vi "Read Teller.vi"(11 "Start Msg Input in":refnum<class "Start Msg Input.lvclass">) -> (2 "Teller":T1 {"Time" format="%<%x %.3X>T"})   [LabVIEW 2020, in "jettl.lvlib" / "Start jettl Msg.lvlib" / "Start Msg Input.lvlib" / "Start Msg Input.lvclass"]
doc: "jettl 6.14.1.98\nNathan Davis - Nathan Davis\nCopyright (c) 2026, Nathan Davis\nMIT"
uses:
  Start Msg Input.lvclass
  Start Msg Input.lvclass/Start Msg Input.ctl
  Relation.ctl
  jettl.lvlib
  Teller Metadata/Teller Metadata.lvclass
  Teller.ctl
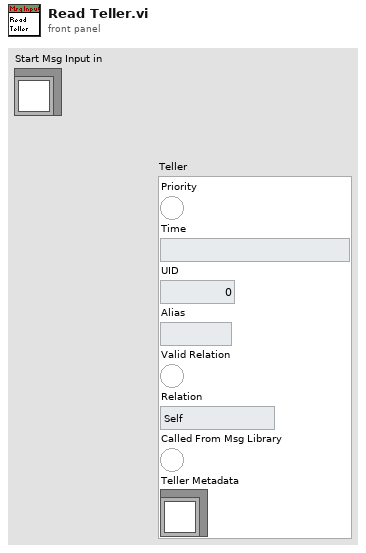
[diagram p1: front panel]
types:
  T1 = typedef "jettl.lvlib/Teller.ctl" = cluster{"Priority":bool, "Time":timestamp, "UID":i32, "Alias":string, "Valid Relation":bool, "Relation":T2, "Called From Msg Library":bool, "Teller Metadata":refnum<class "Teller Metadata.lvclass">}
  T2 = typedef "jettl.lvlib/Relation.ctl" = enum16{"Self", "Parent", "Child"}
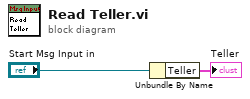
[diagram p0: block diagram]
diagram:
  n1 = Unbundle By Name("Start Msg Input in") -> ("Teller"=→"Teller":T1)
